vi "Read ADC.vi"(8 "error in (no error)":errorcluster, 9 "Canal":u8, 10 "VISA resource name":refnum<visa-resource-name>, 11 "NXP in":refnum<class "NXP.lvclass">) -> (0 "error out":errorcluster, 1 "Response":i32, 2 "VISA resource name 2":refnum<visa-resource-name>, 3 "NXP out":refnum<class "NXP.lvclass">, 4 "String":string)   [LabVIEW 2020, in "NXP.lvclass"]
uses:
  NXP.lvclass
  3fc143b1-23ff-41bf-8ca4-610dcc56367e.vi
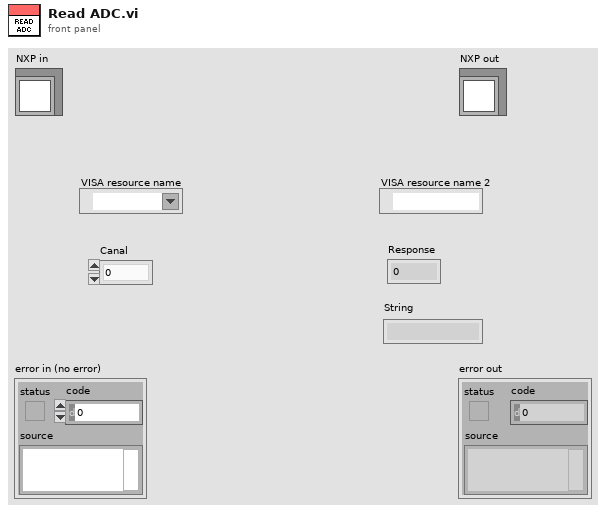
[diagram p1: front panel]
types:
  T1 = enum16{"Write", "Read", "Config", "Reset", "Close"}
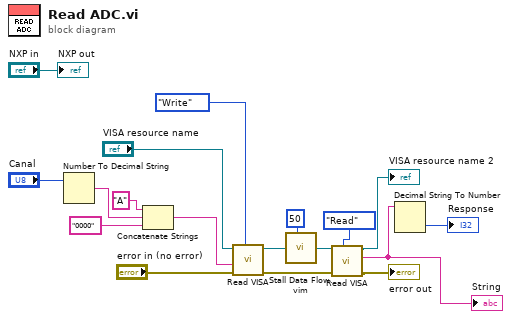
[diagram p0: block diagram]
diagram:
  n1 = Number To Decimal String(number="Canal") -> (decimal integer string=w15:string)  [unwired: 1 in]
  n2 = Concatenate Strings("A" ("string"), w15, "0000" ("string")) -> (w8:string)
  n3 = call "Read VISA.vi"("Opciones"=T1."Write", "error in (no error)"="error in (no error)", "Write"=w8, "VISA com port"="VISA resource name") -> ("error out"=w7:errorcluster, "VISA com port 2"=w6:refnum<visa-resource-name>)  [unwired: 5 in, 1 out]
  n4 = call "Stall Data Flow.vim"("value in"=w6, "milliseconds to wait"=u32 50) -> ("value out"=w5:refnum<visa-resource-name>)  [unwired: 1 out]
  n5 = call "Read VISA.vi"("Opciones"=T1."Read", "error in (no error)"=w7, "VISA com port"=w5) -> ("error out"=→"error out":errorcluster, "Read"=w1:string, "VISA com port 2"=→"VISA resource name 2":refnum<visa-resource-name>)  [unwired: 6 in]
  "String" <- w1
  n6 = Decimal String To Number(string=w1) -> (number=→"Response":i32)  [unwired: 2 in, 1 out]
  "NXP out" <- "NXP in"
